vi "Set PogramState.vi"(4 "Step No.":i32, 5 "End Condition":T1, 6 "Program No.":i32, 7 "Ctrl State":T2, 8 "error in (no error)":errorcluster, 10 "Address (0)":i32, 11 "VISA resource name":refnum<visa-resource-name>) -> (0 "error out":errorcluster, 2 "Status":cluster{"ACK":bool, "Error":bool, "NACK":bool}, 3 "VISA resource name out":refnum<visa-resource-name>)   [LabVIEW 2021, in "Environment Chamber.lvlib" / "Climatic Chamber.lvlib"]
doc: "<b>Program operation control</B>\n\nControls the specified program pattern.\n\n<b>RUN:</b> Starts the specified program pattern. <b>Program No. and Step No. must be specified.</b>\n<b>Pause:</b> Pauses the program operation that is operating.\n<b>Continue:</b> Restarts the paused program operation.\n<b>ADVANCE:</b> Ends the step that is operating and operates the next step.\n<b>END:</b> Ends program operation that is operating at that point, and migrates operation according to the specified end condition. <b>End Condition must be specified</b>"
uses:
  Climatic Chamber.lvlib
  Private/Type Defs/Program CtrlState Enum.ctl
  Private/Type Defs/Program CtrlEndCond Enum.ctl
  Private/Type Defs/Operation_Stop Mode Enum.ctl
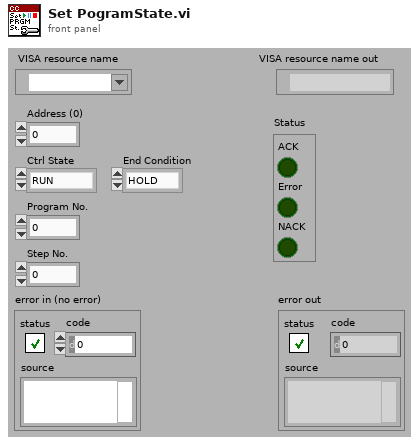
[diagram p1: front panel]
types:
  T1 = typedef "Environment Chamber.lvlib/Climatic Chamber.lvlib/Program CtrlEndCond Enum.ctl" = enum16{"HOLD", "CONST", "OFF", "STANDBY"}
  T2 = typedef "Environment Chamber.lvlib/Climatic Chamber.lvlib/Program CtrlState Enum.ctl" = enum16{"RUN", "PAUSE", "CONTINUE", "ADVANCE", "END"}
  T3 = typedef "Environment Chamber.lvlib/Climatic Chamber.lvlib/Operation_Stop Mode Enum.ctl" = enum16{"RUN", "CONSTANT", "STANDBY", "OFF"}
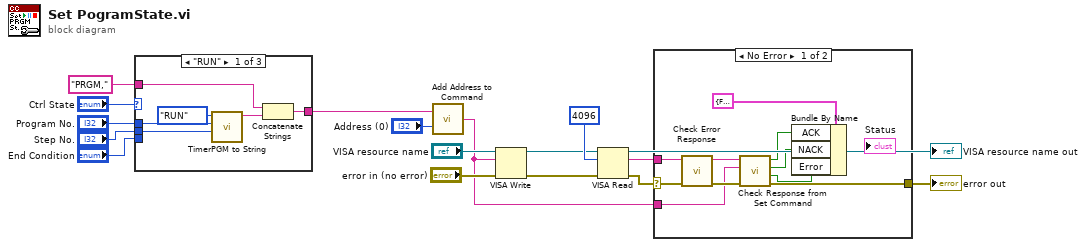
[diagram p0: block diagram]
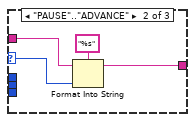
[diagram p2: hidden frame]
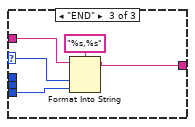
[diagram p3: hidden frame]
diagram:
  n1 = case shown="\"RUN\"" "Ctrl State" {
    selector: "Ctrl State" -> [_ w27 w32]
    tunnel: "Program No." -> [w22 _ _]
    tunnel: "Step No." -> [w21 _ _]
    tunnel: [w19 w26 w31] -> w2
    tunnel: "End Condition" -> [_ _ w30]
    tunnel: "PRGM," -> [w18 w24 w28]
    frame "RUN" {
      n2 = call "TimerPGM to String.vi"("Step No."=w21, "PGM No."=w22, "Op./Stop Mode"=Operation_Stop_Mode_Enum."RUN") -> ("String out"=w20:string)  [unwired: 7 in, 1 out]
      n3 = Concatenate Strings(w18, w20) -> (w19:string)
    }
    frame "PAUSE".."ADVANCE" {
      n4 = Format Into String(format string="%s", initial string=w24, w27) -> (resulting string=w26:string)  [unwired: 1 in, 1 out]
    }
    frame "END" {
      n5 = Format Into String(format string="%s,%s", initial string=w28, w32, w30) -> (resulting string=w31:string)  [unwired: 1 in, 1 out]
    }
  }
  n6 = call "Add Address to Command.vi"("Address (0)"="Address (0)", "Command"=w2) -> ("Command OUT"=w7:string)
  n7 = VISA Write(VISA resource name="VISA resource name", write buffer=w7, error in (no error)="error in (no error)") -> (VISA resource name out=w14:refnum<visa-resource-name>, error out=w13:errorcluster)  [unwired: 1 out]
  n8 = VISA Read(VISA resource name=w14, byte count=u32 4096, error in (no error)=w13) -> (VISA resource name out=→"VISA resource name out":refnum<visa-resource-name>, read buffer=w9:string, error out=w10:errorcluster)  [unwired: 1 out]
  n9 = case shown="No Error" w10 {
    selector: w10 -> [w42 w44]
    tunnel: w9 -> [w43 _]
    tunnel: [w38 w44] -> w8
    tunnel: w7 -> [w39 _]
    frame No Error {
      n10 = call "Check Error Response.vi"("error in (no error)"=w42, "read String"=w43) -> ("error out"=w41:errorcluster, "String out"=w40:string)  [unwired: 7 in, 1 out]
      n11 = call "Check Response from Set Command.vi"("error in (no error)"=w41, "Command"=w39, "Response"=w40) -> ("error out"=w38:errorcluster, "Error"=w33:bool, "NACK"=w34:bool, "ACK"=w35:bool)  [unwired: 5 in]
      n12 = Bundle By Name(cluster=cluster{"ACK":bool, "Error":bool, "NACK":bool} {"ACK"=FALSE, "Error"=FALSE, "NACK"=FALSE} ("Status"), "ACK"=w35, "NACK"=w34, "Error"=w33) -> (→"Status":cluster{"ACK":bool, "Error":bool, "NACK":bool})
    }
    frame Error {
    }
  }
  "error out" <- w8
